vi "Script Setup Advent of Code.vi"   [LabVIEW 2021]
uses:
  <vilib>/LabVIEW Icon API/API_Text.ctl
  <vilib>/LabVIEW Icon API/API_Test Settings.ctl
  <vilib>/LabVIEW Icon API/lv_icon/Controls/Alignment.ctl
  <vilib>/LabVIEW Icon API/API_Text Colors.ctl
  <vilib>/LabVIEW Icon API/LabVIEW Icon API.lvlib
types:
  T1 = typedef "LabVIEW Icon API.lvlib/API_Test Settings.ctl" = cluster{"Font":string, "Alignment":T2, "Size":u8, "Center text":bool, "Capitalize text":bool, "Text color":T3}
  T2 = typedef "Alignment.ctl" = u16
  T3 = typedef "LabVIEW Icon API.lvlib/API_Text Colors.ctl" = cluster{"Line 1 color":u32, "Line 2 color":u32, "Line 3 color":u32, "Line 4 color":u32}
  T4 = typedef "LabVIEW Icon API.lvlib/API_Text.ctl" = cluster{"Line 1 text":string, "Line 2 text":string, "Line 3 text":string, "Line 4 text":string}
  T5 = enum16{"open", "replace", "create", "open or create", "replace or create", "replace or create with confirmation"}
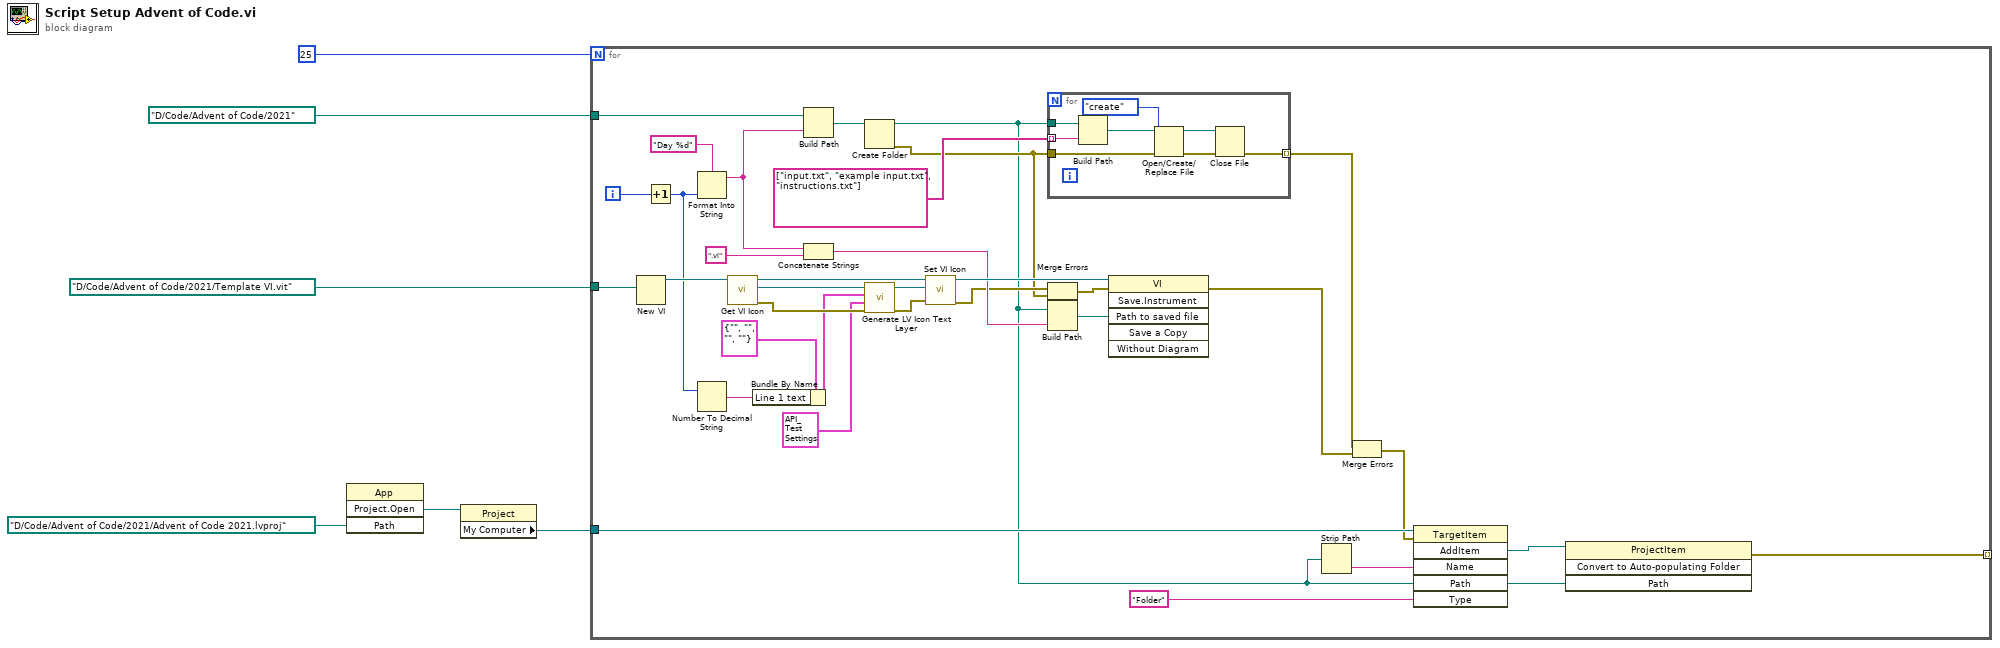
[diagram p0: block diagram]
diagram:
  n1 = invoke class="App" method="Project.Open"("Path"=path "D:/Code/Advent of Code/2021/Advent of Code 2021.lvproj") -> ("Project:Open"=w2:refnum<vi>)  [unwired: 3 in, 3 out]
  n2 = property class="Project"(reference=w2) -> ("My Computer"=w1:refnum<vi>)  [unwired: 1 in, 2 out]
  n3 = for {
    N: 25 -> [_]
    tunnel: path "D:/Code/Advent of Code/2021" ("Advent of Code Folder") -> [w40]
    tunnel: path "D:/Code/Advent of Code/2021/Template VI.vit" -> [w35]
    tunnel: w1 -> [w18]
    tunnel: [w7] -> _ mode=indexing
    i -> [w38]
    n4 = New VI(10:w35) -> (3:w34:refnum<vi>)  [unwired: 6 in, 1 out]
    n5 = Increment(x=w38) -> (x+1=w29:i32)
    n6 = Format Into String(format string="Day %d", w29) -> (resulting string=w17:string)  [unwired: 2 in, 1 out]
    n7 = Number To Decimal String(number=w29) -> (decimal integer string=w27:string)  [unwired: 1 in]
    n8 = call <vilib>:"Get VI Icon.vi"("VI Refnum in"=w34) -> ("error out"=w30:errorcluster, "Icon"=w32:refnum<class "Icon.lvclass">, "VI Refnum out"=w33:refnum<vi>)  [unwired: 8 in]
    n9 = Bundle By Name(cluster=T4 {"Line 1 text"="", "Line 2 text"="", "Line 3 text"="", "Line 4 text"=""} ("Text"), "Line 1 text"=w27) -> (w26:T4)
    n10 = Build Path(base path=w40, name or relative path=w17) -> (appended path=w37:path)
    n11 = Concatenate Strings(w17, ".vi" ("string")) -> (w21:string)
    n12 = Create Folder(path (use dialog)=w37) -> (created path=w8:path, error out=w11:errorcluster)  [unwired: 2 in, 1 out]
    n13 = call <vilib>:"Generate LV Icon Text Layer.vi"("error in (no error)"=w30, "Text settings"=T1 {"Font"="Small Fonts", "Alignment"=0, "Size"=15, "Center text"=TRUE, "Capitalize text"=TRUE, "Text color"={"Line 1 color"=0, "Line 2 color"=0, "Line 3 color"=0, "Line 4 color"=0}}, "Text"=w26, "Icon in"=w32) -> ("error out"=w24:errorcluster, "Icon out"=w31:refnum<class "Icon.lvclass">)  [unwired: 6 in]
    n14 = call <vilib>:"Set VI Icon.vi"("error in (no error)"=w24, "Icon"=w31, "VI Refnum in"=w33) -> ("error out"=w19:errorcluster, "VI Refnum out"=w23:refnum<vi>)  [unwired: 7 in]
    n15 = for {
      tunnel: w8 -> [w48]
      tunnel: string[] ["input.txt", "example input.txt", "instructions.txt"] -> [w47] mode=indexing
      tunnel: w11 -> [w43]
      tunnel: [w42] -> w15 mode=indexing
      n16 = Build Path(base path=w48, name or relative path=w47) -> (appended path=w46:path)
      n17 = Open/Create/Replace File(file path (use dialog)=w46, error in=w43, operation (0:open)=T5."create") -> (refnum out=w45:refnum<file>, error out=w44:errorcluster)  [unwired: 3 in, 1 out]
      n18 = Close File(refnum=w45, error in=w44) -> (error out=w42:errorcluster)  [unwired: 1 out]
    }
    n19 = Merge Errors(w19, w11) -> (w12:errorcluster)
    n20 = Build Path(base path=w8, name or relative path=w21) -> (appended path=w20:path)
    n21 = invoke class="VI" method="Save.Instrument"(reference=w23, error in=w12, "Path to saved file"=w20) -> (error out=w14:errorcluster)  [unwired: 3 in, 5 out]
    n22 = Strip Path(path=w8) -> (name=w10:string)  [unwired: 1 out]
    n23 = Merge Errors(w15, w14) -> (w13:errorcluster)
    n24 = invoke class="TargetItem" method="AddItem"(reference=w18, error in=w13, "Name"=w10, "Path"=w8, "Type"="Folder") -> ("AddItem"=w9:refnum<vi>)  [unwired: 1 in, 5 out]
    n25 = invoke class="ProjectItem" method="Convert to Auto-populating Folder"(reference=w9, "Path"=w8) -> (error out=w7:errorcluster)  [unwired: 2 in, 3 out]
  }
